vi "openbci_startup.vi"(8 "error in":errorcluster, 11 "OBCI dev in":T1={"COM port"="", "n_ch (8)"=enum."8 Channels", "delay_tx"=50}) -> (0 "error out":errorcluster, 2 "start_up_string":string, 3 "OBCI dev out":T1={"COM port"="", "n_ch (8)"=enum."8 Channels", "delay_tx"=50})   [LabVIEW 2013]
doc: "Serial Setup for OpenBCI V3\n\nDefault 115200bps 8-N-1\nTimeOut 5 seconds"
uses:
  Control Def/openbci_device.ctl
  Control Def/channel_count.ctl
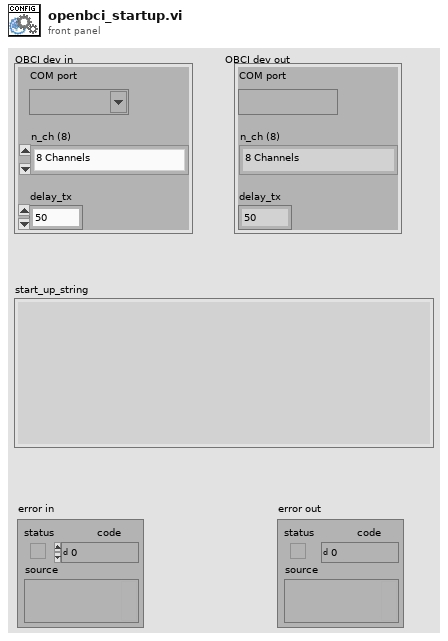
[diagram p1: front panel]
types:
  T1 = typedef "openbci_device.ctl" = cluster{"COM port":refnum<visa-resource-name>, "n_ch (8)":T2, "delay_tx":u32}
  T2 = typedef "channel_count.ctl" = enum16{"8 Channels", "16 Channels"}
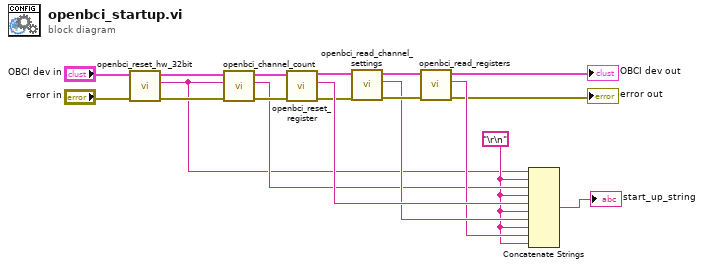
[diagram p0: block diagram]
diagram:
  w2 = "\r\n"
  n1 = call "openbci_reset_hw_32bit.vi"("error in (no error)"="error in", "OBCI dev in"="OBCI dev in") -> ("error out"=w4:errorcluster, "reset_str"=w1:string, "OBCI dev out"=w5:T1)  [unwired: 7 in]
  n2 = call "openbci_channel_count.vi"("error in (no error)"=w4, "reset_str_in"=w1, "OBCI dev in"=w5) -> ("error out"=w18:errorcluster, "str_out"=w3:string, "OBCI dev out"=w17:T1)  [unwired: 6 in]
  n3 = call "openbci_reset_register.vi"("error in (no error)"=w18, "OBCI dev in"=w17) -> ("error out"=w14:errorcluster, "reset_reg_str"=w16:string, "OBCI dev out"=w15:T1)  [unwired: 7 in]
  n4 = call "openbci_read_channel_settings.vi"("error in (no error)"=w14, "OBCI dev in"=w15) -> ("error out"=w13:errorcluster, "channel_default_config"=w11:string, "OBCI dev out"=w12:T1)  [unwired: 7 in]
  n5 = call "openbci_read_registers.vi"("error in (no error)"=w13, "OBCI dev in"=w12) -> ("error out"=→"error out":errorcluster, "registers"=w10:string, "OBCI dev out"=→"OBCI dev out":T1)  [unwired: 7 in]
  n6 = Concatenate Strings(w1, w2, w3, w2, w16, w2, w11, w2, w10, w2) -> (→"start_up_string":string)
